vi "count rate.vi"() -> ()   [LabVIEW 2016, in "Top Level.lvlib"]
uses:
  Top Level.lvlib
panel:
  out "error out":errorcluster
  in  "stop":bool
  out "count rate(cps)":dbl
  out "Waveform Chart":dbl(graph)
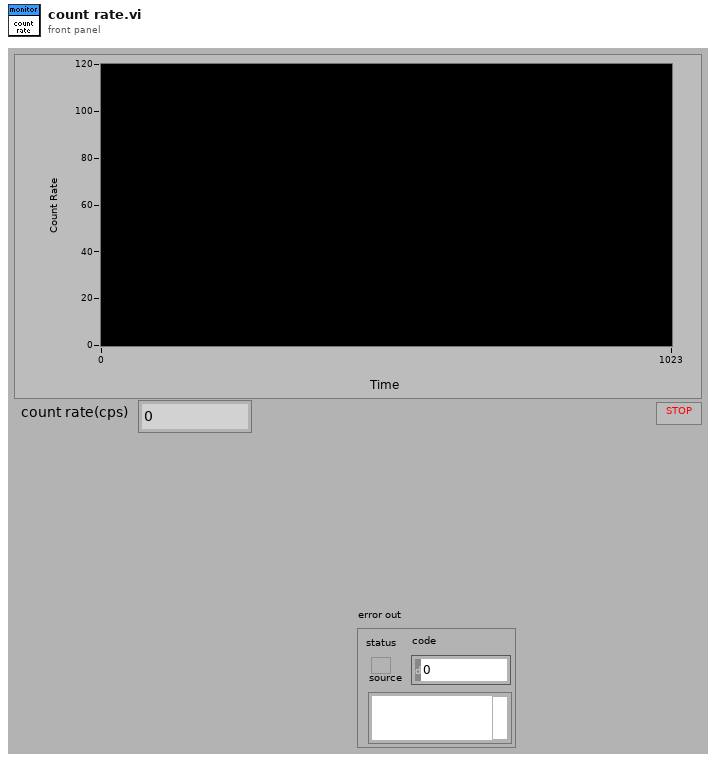
[diagram p1: front panel]
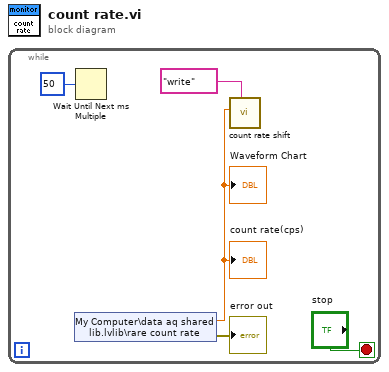
[diagram p0: block diagram]
diagram:
  n1 = while {
    stop <- "stop" stop-if-true
    n2 = shared-variable "My Computer\\data aq shared lib.lvlib\\rare count rate"() -> (w2:dbl, error out=→"error out":errorcluster)  [unwired: 1 in]
    "Waveform Chart" <- w2
    "count rate(cps)" <- w2
    n3 = Wait Until Next ms Multiple(millisecond multiple=u32 50) -> ()  [unwired: 1 out]
    n4 = call "count rate shift.vi"("read or write"="write" ("Combo Box"), "count rate in"=w2) -> ()  [unwired: 9 in, 1 out]
  }
